vi "SENS_OFFS_DIV.vi"(0 "VISA IN":refnum<visa-resource-name>, 1 "Divisor Value":i32, 5 "error in":errorcluster, 7 "Channel":i32) -> (14 "VISA Out":refnum<visa-resource-name>, 19 "error out":errorcluster)   [LabVIEW 2018, in "PNA-X.lvlib"]
doc: "SENSe<cnum>:OFFSet:DIVisor <num> \n1790\n\n(Read-Write) Specifies (along with the multiplier) the value to multiply by the stimulus. \nParameters \n<cnum> Any existing channel number. If unspecified, value is set to 1 \n<num> Divisor value. Range is 1 to 1000 \nExamples SENS:OFFS:DIV 3 \nsense2:offset:divisor 2 \nQuery Syntax SENSe<cnum>:OFFSet:DIVisor? \nReturn Type Numeric \nDefault 1"
uses:
  PNA-X.lvlib
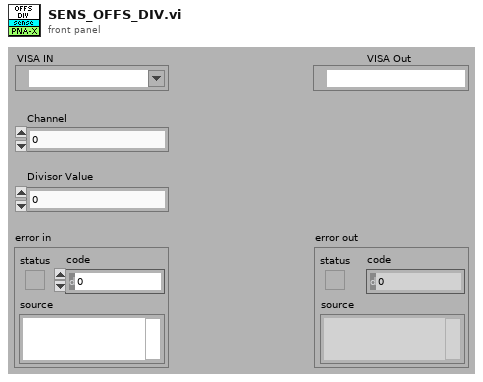
[diagram p1: front panel]
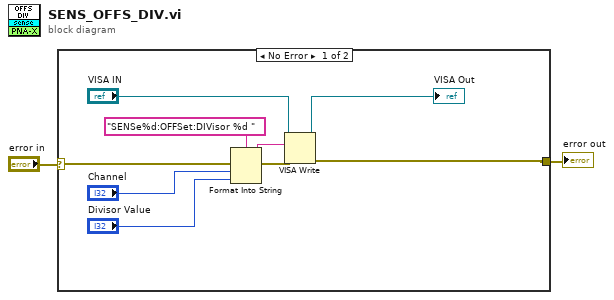
[diagram p0: block diagram]
diagram:
  n1 = case shown="No Error" "error in" {
    selector: "error in" -> [w11 w12]
    tunnel: [w6 w12] -> w1
    frame No Error {
      n2 = Format Into String(format string="SENSe%d:OFFSet:DIVisor %d " ("Cmdline"), error in=w11, "Channel", "Divisor Value") -> (resulting string=w9:string, error out=w10:errorcluster)  [unwired: 1 in]
      n3 = VISA Write(VISA resource name="VISA IN", write buffer=w9, error in (no error)=w10) -> (VISA resource name out=→"VISA Out":refnum<visa-resource-name>, error out=w6:errorcluster)  [unwired: 1 out]
    }
    frame Error {
    }
  }
  "error out" <- w1
